vi "Complete Pattern Script_SPI.vi"(6 "SPI_Mode":T1, 8 "error in (no error)":errorcluster, 9 "Pattern Contents":string, 10 "Pattern Name":string, 11 "DigiPattern_Generator.lvclass":refnum<class "DigiPattern_Generator.lvclass">) -> (0 "error out":errorcluster, 2 "All Pattern Script out":string, 3 "DigiPattern_Generator.lvclass out":refnum<class "DigiPattern_Generator.lvclass">)   [LabVIEW 2018, in "DigiPattern_Generator.lvclass"]
uses:
  DigiPattern_Generator.lvclass
  SPI/Config Read SPI/SPI_Mode.ctl
  BML_Frame_Root/BML_Frame_Root.lvclass
  SPI/Config Read SPI/Config_Read_SPI.lvclass
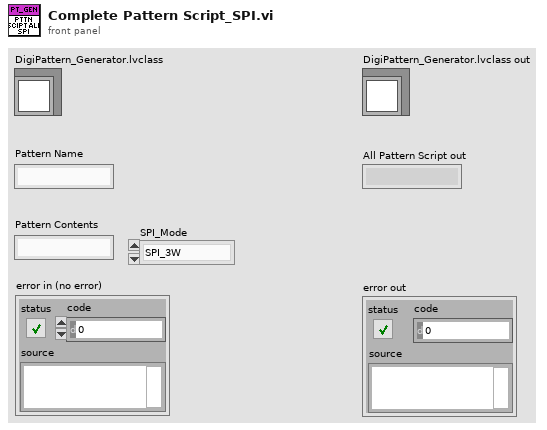
[diagram p1: front panel]
types:
  T1 = typedef "Config_Read_SPI.lvclass/SPI_Mode.ctl" = enum16{"SPI_3W", "SPI_4W"}
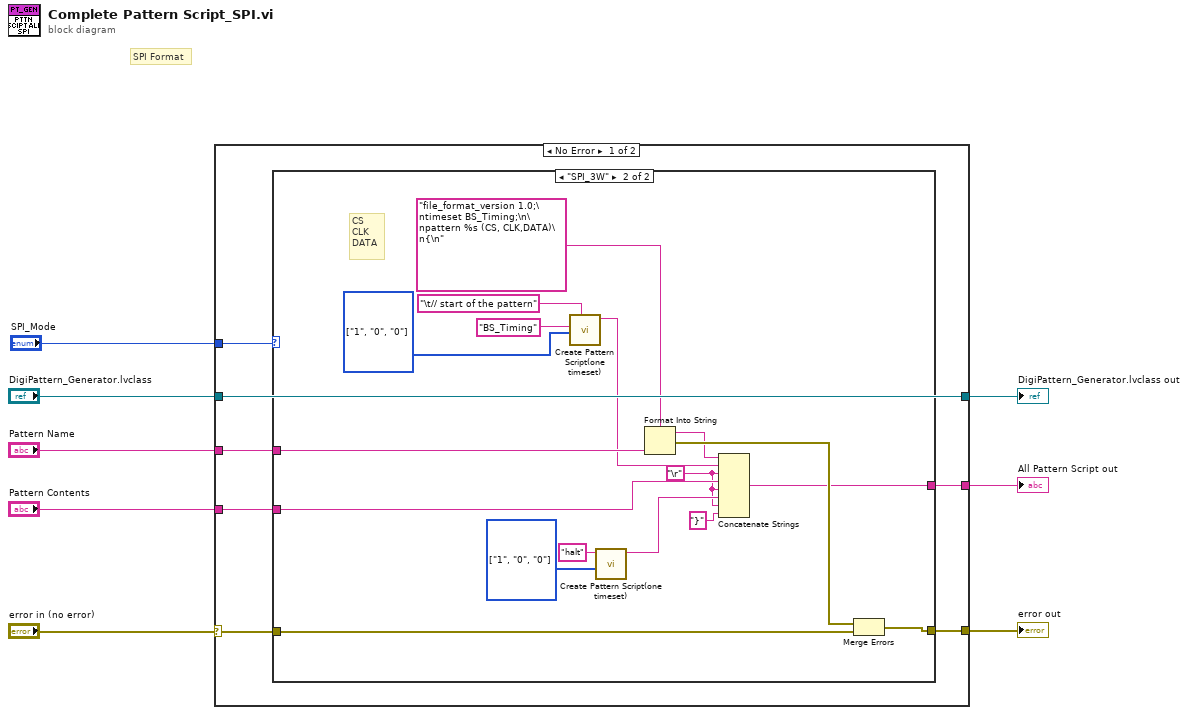
[diagram p0: block diagram]
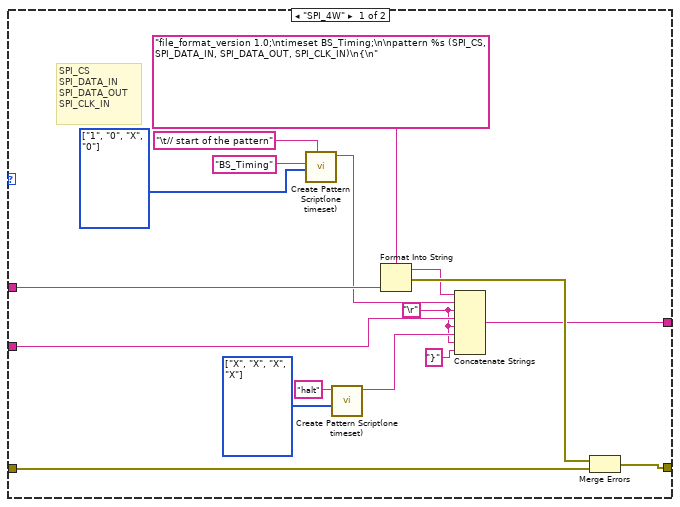
[diagram p2: hidden frame]
diagram:
  # "SPI Format"
  n1 = case shown="No Error" "error in (no error)" {
    selector: "error in (no error)" -> [w13 w51]
    tunnel: "DigiPattern_Generator.lvclass" -> [w11 w50]
    tunnel: [w12 w51] -> w6
    tunnel: [w11 w50] -> w5
    tunnel: "Pattern Name" -> [w15 _]
    tunnel: "Pattern Contents" -> [w14 _]
    tunnel: [w10 _] -> w2
    tunnel: "SPI_Mode" -> [w9 _]
    frame No Error {
      n2 = case shown="\"SPI_3W\"" w9 {
        tunnel: w15 -> [w32 w49]
        tunnel: w14 -> [w31 w48]
        tunnel: w13 -> [w29 w46]
        tunnel: [w28 w45] -> w12
        tunnel: [w27 w44] -> w10
        frame "SPI_4W" {
          w16 = enum16{"0", "1", "L", "H", "X", "V", "D", "M"}[] [enum."X", enum."X", enum."X", enum."X"] items=["0", "1", "L", "H", "X", "V", "D", "M"] ("PinState")
          w17 = enum16{"0", "1", "L", "H", "X", "V", "D", "M"}[] [enum."1", enum."0", enum."X", enum."0"] items=["0", "1", "L", "H", "X", "V", "D", "M"] ("PinState")
          w20 = "\r"
          # "SPI_CS\nSPI_DATA_IN\nSPI_DATA_OUT\nSPI_CLK_IN"
          n3 = call "Create Pattern Script(one timeset).vi"("Notes"="\t// start of the pattern", "PinState"=w17, "timeset name"="BS_Timing") -> ("string out"=w23:string)  [unwired: 8 in]
          n4 = call "Create Pattern Script(one timeset).vi"("PinState"=w16, "opcode"="halt") -> ("string out"=w22:string)  [unwired: 9 in]
          n5 = Format Into String(format string="file_format_version 1.0;\ntimeset BS_Timing;\n\npattern %s (SPI_CS, SPI_DATA_IN, SPI_DATA_OUT, SPI_CLK_IN)\n{\n", w32) -> (resulting string=w24:string, error out=w30:errorcluster)  [unwired: 2 in]
          n6 = Concatenate Strings(w24, w23, w20, w31, w20, w22, w20, "}") -> (w27:string)
          n7 = Merge Errors(w30, w29) -> (w28:errorcluster)
        }
        frame "SPI_3W" {
          w33 = enum16{"0", "1", "L", "H", "X", "V", "D", "M"}[] [enum."1", enum."0", enum."0"] items=["0", "1", "L", "H", "X", "V", "D", "M"] ("PinState")
          w34 = enum16{"0", "1", "L", "H", "X", "V", "D", "M"}[] [enum."1", enum."0", enum."0"] items=["0", "1", "L", "H", "X", "V", "D", "M"] ("PinState")
          w37 = "\r"
          # "CS\nCLK\nDATA"
          n8 = call "Create Pattern Script(one timeset).vi"("Notes"="\t// start of the pattern", "PinState"=w34, "timeset name"="BS_Timing") -> ("string out"=w40:string)  [unwired: 8 in]
          n9 = call "Create Pattern Script(one timeset).vi"("PinState"=w33, "opcode"="halt") -> ("string out"=w39:string)  [unwired: 9 in]
          n10 = Format Into String(format string="file_format_version 1.0;\ntimeset BS_Timing;\n\npattern %s (CS, CLK,DATA)\n{\n", w49) -> (resulting string=w41:string, error out=w47:errorcluster)  [unwired: 2 in]
          n11 = Concatenate Strings(w41, w40, w37, w48, w37, w39, w37, "}") -> (w44:string)
          n12 = Merge Errors(w47, w46) -> (w45:errorcluster)
        }
      }
    }
    frame Error {
    }
  }
  "error out" <- w6
  "DigiPattern_Generator.lvclass out" <- w5
  "All Pattern Script out" <- w2
